vi "System Startup.vi"(8 "error in (no error)":errorcluster, 10 "StatusStr ref":refnum<vi>, 11 "Application in":refnum<class "Application.lvclass">) -> (0 "error out":errorcluster, 3 "Application out":refnum<class "Application.lvclass">)   [LabVIEW 2019, in "Application.lvclass"]
doc: "Developed by Kevin Thompson\nkevin@thompsonengineering.net\n\nCopyright 2018-2020\nThompson Engineering, LLC"
uses:
  Application.lvclass
  Subsystems/Config/Config.lvclass
  DataTypes/Dependency--cluster.ctl
  Subsystems/Main/Main.lvclass
  Common/ErrorHandler/ErrorHandler.lvclass
  Subsystems/DAQ_Engine/DAQ_Engine.lvclass
  Subsystems/Log_Engine/Log_Engine.lvclass
  Common/DataTypes/TD GetSet ActionSelect--enum.ctl
  Common/DataQ_SE/TD MeasData--cluster.ctl
  Common/DataTypes/InverterPhaseData--cluster.ctl
  Application.lvclass/Application.ctl
  Accessors/Set Dependency.vi
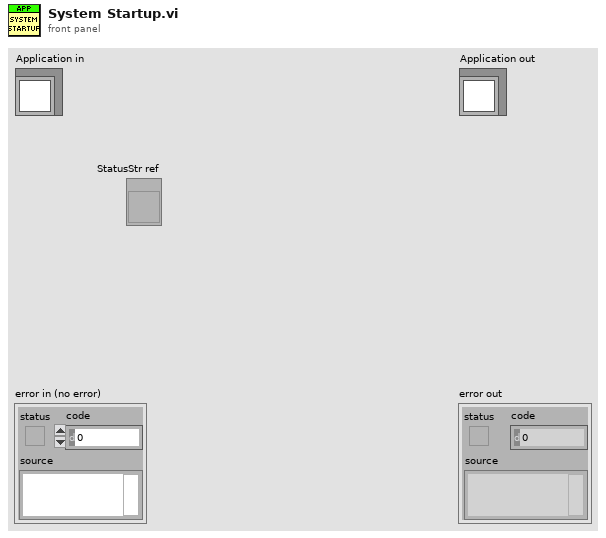
[diagram p1: front panel]
types:
  T1 = typedef "TD GetSet ActionSelect--enum.ctl" = enum16{"Init", "Get", "Set"}
  T2 = typedef "Application.lvclass/Dependency--cluster.ctl" = cluster{"Config":refnum<class "Config.lvclass">, "Main":refnum<class "Main.lvclass">, "ErrorHandler":refnum<class "ErrorHandler.lvclass">, "DAQ_Engine":refnum<class "DAQ_Engine.lvclass">, "Log_Engine":refnum<class "Log_Engine.lvclass">}
  T3 = typedef "TD MeasData--cluster.ctl" = cluster{"Timestamp":timestamp, "ESR_Ohm":dbl[], "DUT data":T4[], "DUT INVERTER data":cluster{"Raw ESR sum":dbl, "scaled raw ESR sum":dbl, "scaled and averaged raw ESR sum":dbl, "Total power":dbl}[]}
  T4 = typedef "InverterPhaseData--cluster.ctl" = cluster{"RawESR_Ohm":dbl, "TcompAvgESR_Ohm":dbl, "VoutRMS_V":dbl, "IoutRMS_A":dbl, "PF":dbl, "AvgPF":dbl, "Power_W":dbl, "AvgPower_W":dbl, "efficiency":dbl}
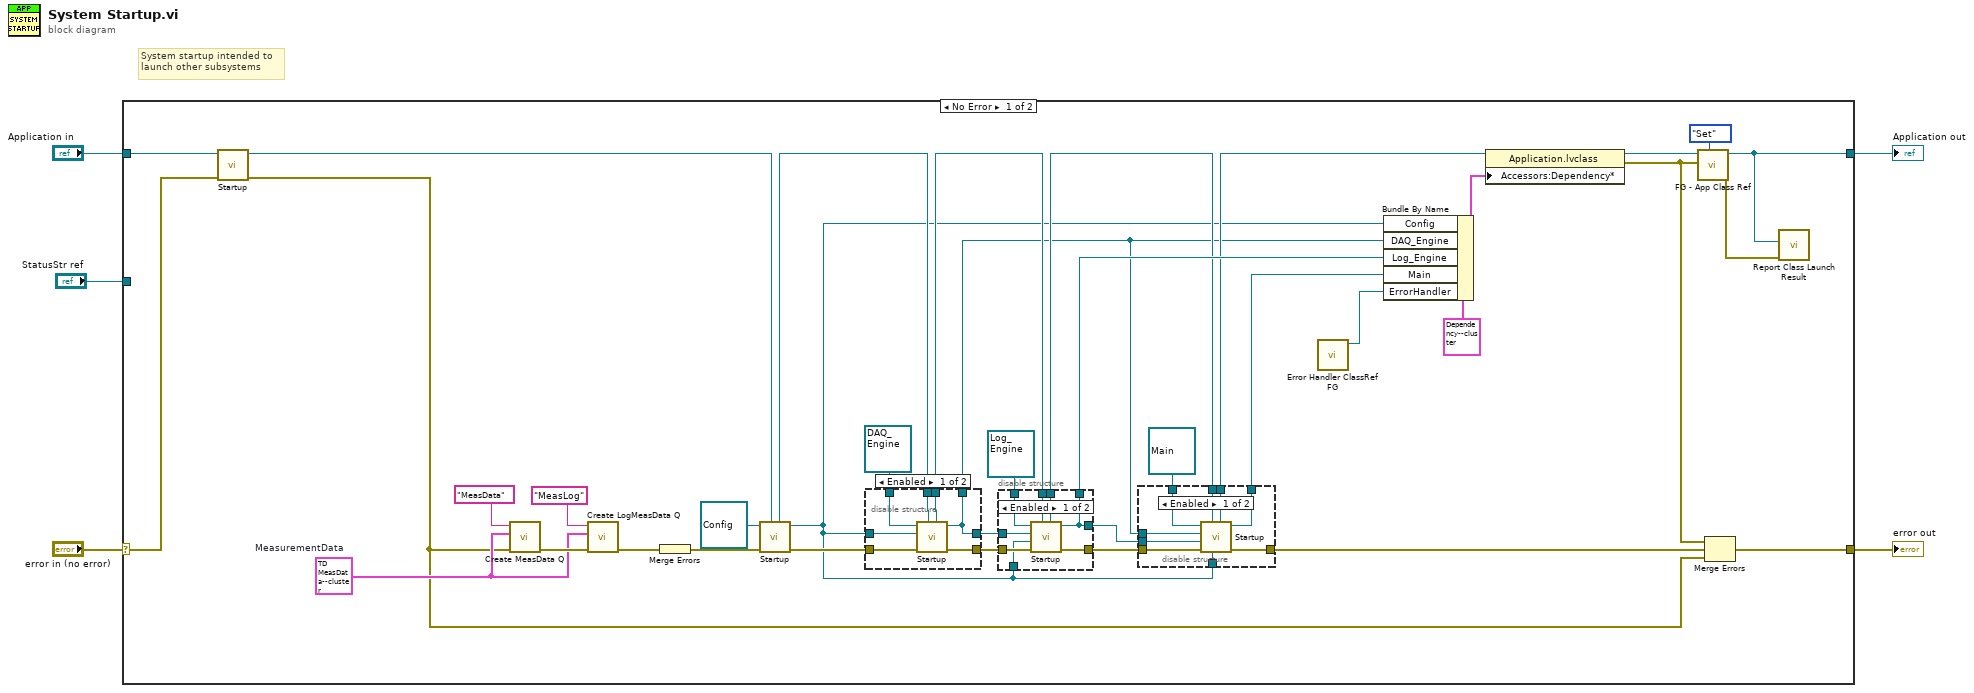
[diagram p0: block diagram]
diagram:
  # "System startup intended to\nlaunch other subsystems"
  n1 = case shown="No Error" "error in (no error)" {
    selector: "error in (no error)" -> [w8 w74]
    tunnel: [w42 w74] -> w4
    tunnel: [w41 w73] -> w2
    tunnel: "Application in" -> [w9 w73]
    tunnel: "StatusStr ref" -> [_ _]
    frame No Error {
      w27 = T3 {"Timestamp"=timestamp(0 s since 1904-01-01), "ESR_Ohm"=[], "DUT data"=[], "DUT INVERTER data"=[]}  # MeasurementData
      n2 = call "Startup.vi"("error in (no error)"=w8, "Application in"=w9) -> ("error out"=w7:errorcluster, "Application out"=w6:refnum<class "Application.lvclass">)  [unwired: 8 in]
      n3 = call "Create MeasData Q.vi"("error in (no error)"=w7, "MeasurementData"=w27, "QName"="MeasData") -> ("error out"=w28:errorcluster)  [unwired: 7 in, 1 out]
      n4 = call "Create LogMeasData Q.vi"("error in (no error)"=w28, "MeasData"=w27, "QName"="MeasLog") -> ("error out"=w26:errorcluster)  [unwired: 7 in, 1 out]
      n5 = Merge Errors(w26) -> (w24:errorcluster)
      n6 = call "Startup.vi"("Application in"=w6, "error in (no error)"=w24, "Config in"=refnum<class "Config.lvclass"> refnum) -> ("error out"=w39:errorcluster, "Config out"=w11:refnum<class "Config.lvclass">, "Application out"=w25:refnum<class "Application.lvclass">)  [unwired: 6 in]
      n7 = disable-structure shown="Enabled" {
        disable-tunnel: w39 -> [w70 w72]
        disable-tunnel: [w69 w72] -> w23
        disable-tunnel: w25 -> [w68 _]
        disable-tunnel: [w64 w71] -> w14
        disable-tunnel: w11 -> [w67 _]
        disable-tunnel: refnum<class "DAQ_Engine.lvclass"> refnum ("DAQ_Engine.lvclass") -> [w66 w71]
        disable-tunnel: [w65 _] -> w16
        disable-tunnel: [w64 _] -> w22
        frame Enabled {
          n8 = call "Startup.vi"("Application"=w68, "error in (no error)"=w70, "Config"=w67, "DAQ_Engine in"=w66) -> ("error out"=w69:errorcluster, "DAQ_Engine out"=w64:refnum<class "DAQ_Engine.lvclass">, "Application out"=w65:refnum<class "Application.lvclass">)  [unwired: 5 in]
        }
        frame Disabled {
        }
      }
      n9 = disable-structure shown="Enabled" {
        disable-tunnel: [w50 w51] -> w13
        disable-tunnel: w23 -> [w49 w51]
        disable-tunnel: refnum<class "Log_Engine.lvclass"> refnum ("Log_Engine.lvclass") -> [w48 w52]
        disable-tunnel: w16 -> [w47 _]
        disable-tunnel: w11 -> [w46 _]
        disable-tunnel: w22 -> [w45 _]
        disable-tunnel: [w43 w52] -> w21
        disable-tunnel: [w44 _] -> w15
        disable-tunnel: [w43 _] -> w10
        frame Enabled {
          n10 = call "Startup.vi"("Application"=w47, "error in (no error)"=w49, "Config"=w46, "DAQ_Engine"=w45, "Log_Engine in"=w48) -> ("error out"=w50:errorcluster, "Log_Engine out"=w43:refnum<class "Log_Engine.lvclass">, "Application out"=w44:refnum<class "Application.lvclass">)  [unwired: 4 in]
        }
        frame Disabled {
        }
      }
      n11 = disable-structure shown="Enabled" {
        disable-tunnel: w13 -> [w61 w63]
        disable-tunnel: [w60 w63] -> w31
        disable-tunnel: w15 -> [w59 _]
        disable-tunnel: [w58 _] -> w17
        disable-tunnel: [w57 w62] -> w18
        disable-tunnel: refnum<class "Main.lvclass"> refnum ("Main.lvclass") -> [w56 w62]
        disable-tunnel: w14 -> [w55 _]
        disable-tunnel: w11 -> [w54 _]
        disable-tunnel: w10 -> [w53 _]
        frame Enabled {
          n12 = call "Startup.vi"("Config"=w54, "Application"=w59, "error in (no error)"=w61, "Log_Engine"=w53, "DAQ_Engine"=w55, "Main in"=w56) -> ("error out"=w60:errorcluster, "Main out"=w57:refnum<class "Main.lvclass">, "Application out"=w58:refnum<class "Application.lvclass">)  [unwired: 3 in]
        }
        frame Disabled {
        }
      }
      n13 = call "Error Handler ClassRef FG.vi"() -> ("ErrorHandler out"=w36:refnum<class "ErrorHandler.lvclass">)  [unwired: 10 in, 1 out]
      n14 = Bundle By Name(cluster=T2 {"Config"=refnum, "Main"=refnum, "ErrorHandler"=refnum, "DAQ_Engine"=refnum, "Log_Engine"=refnum} ("Dependency"), "Config"=w11, "DAQ_Engine"=w14, "Log_Engine"=w21, "Main"=w18, "ErrorHandler"=w36) -> (w38:T2)
      n15 = property class="Application.lvclass"(reference=w17, "Accessors:Dependency*"=w38) -> (reference out=w35:refnum<class "Application.lvclass">, error out=w34:errorcluster)  [unwired: 1 in]
      n16 = call "FG - App Class Ref.vi"("Application in"=w35, "error in (no error)"=w34, "action (Get)"=TD_GetSet_ActionSelect--enum."Set") -> ("Application out"=w41:refnum<class "Application.lvclass">, "error out"=w33:errorcluster)  [unwired: 6 in]
      n17 = Merge Errors(w34, w31, w7) -> (w42:errorcluster)
      n18 = call "Report Class Launch Result.vi"("Object"=w41, "error in (no error)"=w33) -> ()  [unwired: 8 in, 1 out]
    }
    frame Error {
    }
  }
  "error out" <- w4
  "Application out" <- w2
